vi "Firmware Wizard Check INI.vi"(8 "Error In":errorcluster) -> (0 "Error Out":errorcluster)   [LabVIEW 2014, in "LMH-LINX.lvlib"]
uses:
  <vilib>/MakerHub/LINX/LMH-LINX.lvlib
  <vilib>/Utility/config.llb/Write Key (Path).vi
  <vilib>/MakerHub/Toolbox/LMH-Toolbox.lvlib
  <vilib>/Utility/config.llb/NI_LVConfig.lvlib
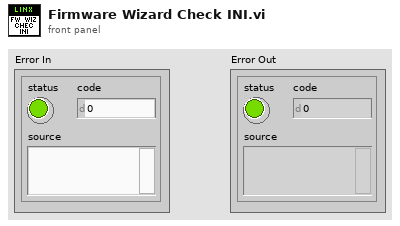
[diagram p1: front panel]
types:
  T1 = typedef "NI_LVConfig.lvlib/Config Data RefNum.ctl" = refnum<k1>
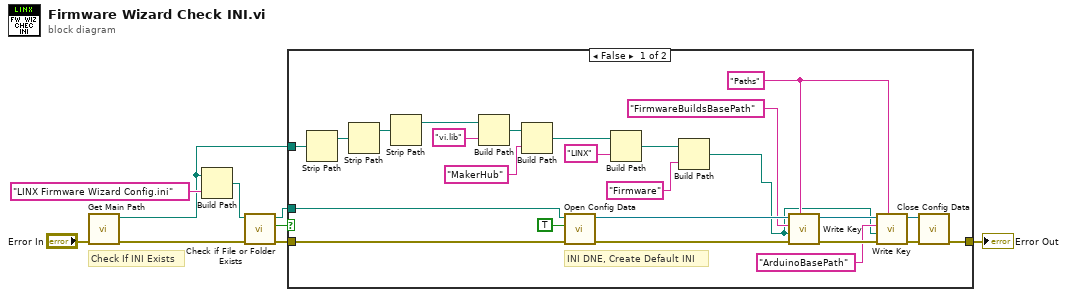
[diagram p0: block diagram]
diagram:
  # "Check If INI Exists"
  n1 = call <vilib>:"Get Main Path.vi"("Error In"="Error In") -> ("Error Out"=w9:errorcluster, "Main Dir"=w2:path)  [unwired: 8 in, 1 out]
  n2 = Build Path(base path=w2, name or relative path="LINX Firmware Wizard Config.ini") -> (appended path=w6:path)
  n3 = call <vilib>:"Check if File or Folder Exists.vi"("error in (no error)"=w9, "path"=w6) -> ("error out"=w5:errorcluster, "file or folder exists?"=w4:bool, "dup path"=w1:path)  [unwired: 7 in]
  n4 = case shown="False" w4 {
    tunnel: w5 -> [w30 w35]
    tunnel: [w27 w35] -> w3
    tunnel: w2 -> [w29 _]
    tunnel: w1 -> [w26 _]
    frame False {
      w14 = "Paths" ("section")
      # "INI DNE, Create Default INI"
      n5 = Strip Path(path=w29) -> (stripped path=w25:path)  [unwired: 1 out]
      n6 = Strip Path(path=w25) -> (stripped path=w24:path)  [unwired: 1 out]
      n7 = Strip Path(path=w24) -> (stripped path=w23:path)  [unwired: 1 out]
      n8 = Build Path(base path=w23, name or relative path="vi.lib") -> (appended path=w21:path)
      n9 = Build Path(base path=w21, name or relative path="MakerHub") -> (appended path=w19:path)
      n10 = call <vilib>:"Open Config Data.vi"("error in (no error)"=w30, "create file if necessary (T)"=TRUE, "configuration file path"=w26) -> ("error out"=w34:errorcluster, "refnum"=w33:T1)  [unwired: 6 in, 1 out]
      n11 = Build Path(base path=w19, name or relative path="LINX") -> (appended path=w17:path)
      n12 = Build Path(base path=w17, name or relative path="Firmware") -> (appended path=w12:path)
      n13 = call-poly <vilib>:"Write Key.vi"("section"=w14, "error in (no error)"=w34, "value"=w12, "key"="FirmwareBuildsBasePath", "refnum"=w33) -> ("error out"=w15:errorcluster, "refnum out"=w16:T1)  [unwired: 4 in, 1 out]
      n14 = call-poly <vilib>:"Write Key.vi"("section"=w14, "error in (no error)"=w15, "value"=w12, "key"="ArduinoBasePath", "refnum"=w16) -> ("error out"=w10:errorcluster, "refnum out"=w11:T1)  [unwired: 4 in, 1 out]
      n15 = call <vilib>:"Close Config Data.vi"("error in (no error)"=w10, "refnum"=w11) -> ("error out"=w27:errorcluster)  [unwired: 8 in, 1 out]
    }
    frame True {
      # "INI Exists, Nothing To Do"
    }
  }
  "Error Out" <- w3
